vi "Projectile_Motion_2D.vi"() -> ()   [LabVIEW 2017]
panel:
  in  "Number of Particles":i32=100
  in  "Power of Force":dbl[](array[numeric])
  out "Initial Velocity":dbl[][](array[numeric])
  out "Initial Position":dbl[][](array[numeric])
  in  "Acceleration":dbl[](array[numeric])
  out "XY Graph":cluster{dbl[], dbl[]}(graph)
  in  "stop":bool
  # "IMPORTANT: The Power of force\nand the acceleration MUST be initialized\nso that the program can run. Default\nvalues for power are 1 and 1. Default\nvalues for acceleration are 0 (x direction) and\n-1 (y direction, acting like gravity).  The central\nforce term is more evident when acceleration is\nchosen to be 0 and 0 in both directions"
  # "Details: This program creates a choosen amount of\nparticles in random positions from\n-10 < position < 10 and random velocities\nfrom 0 < velocity < 1 and plots their motion. \nParticles are subjected to acceleration,\nspecular reflection once it hits a wall boundary, a \ndrag term that is veocity dependent and \na central force term whose power can be controlled by\nthe user."
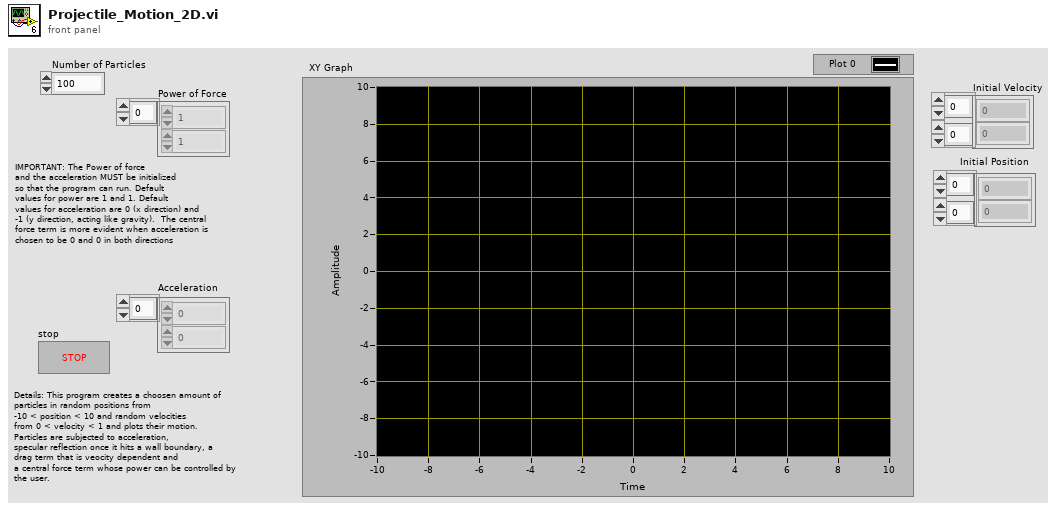
[diagram p1: front panel]
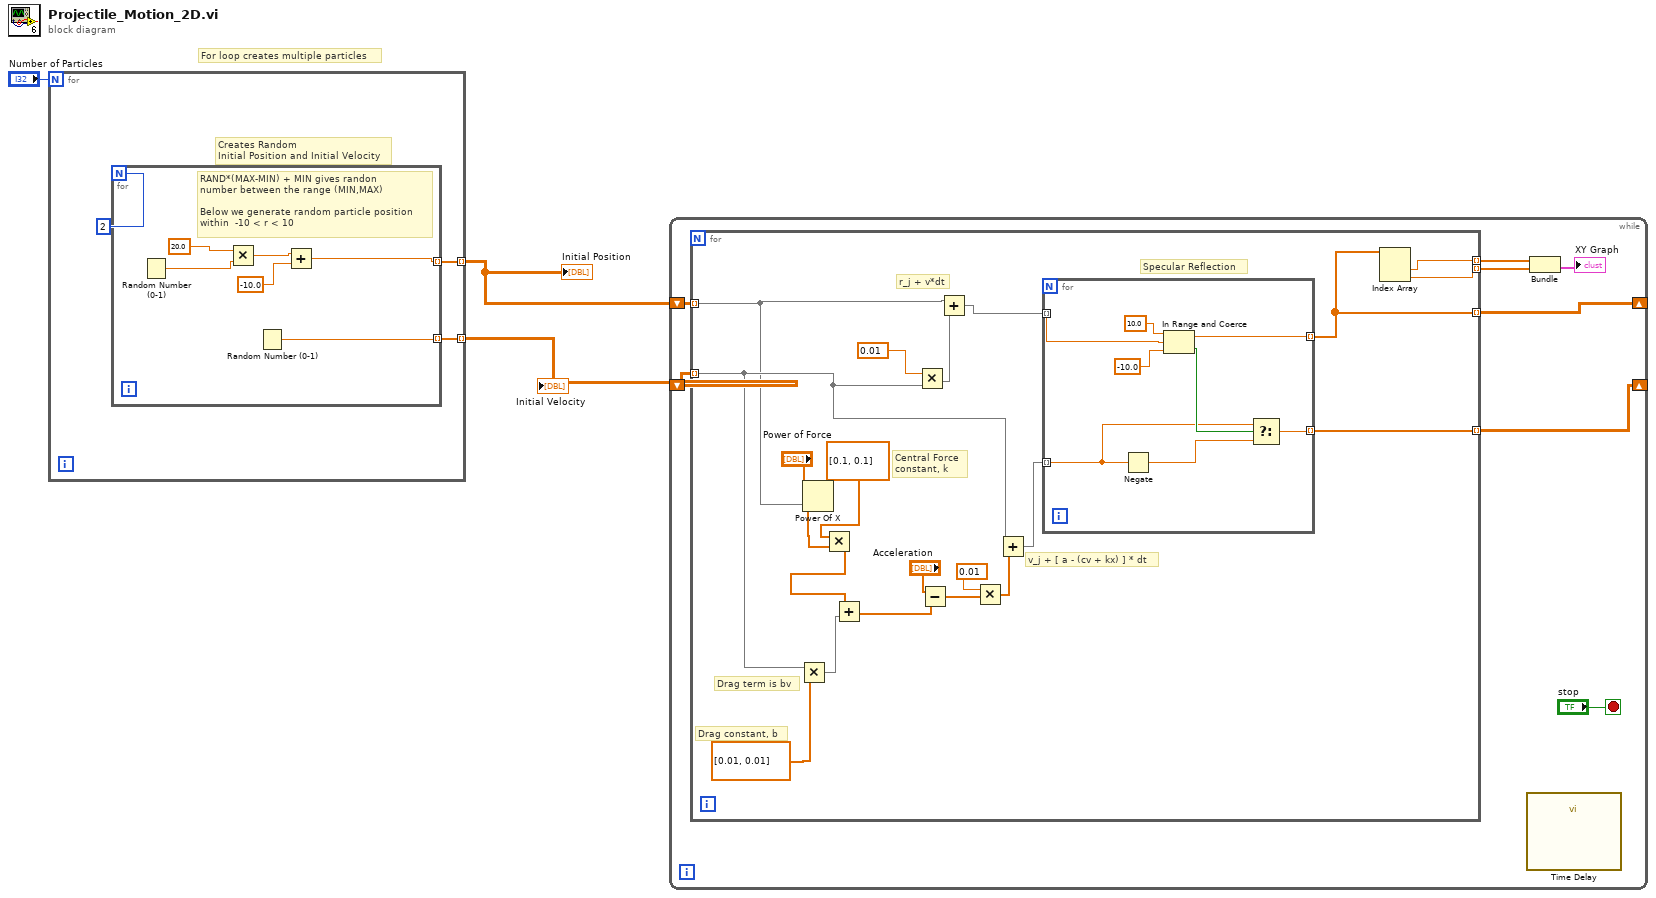
[diagram p0: block diagram]
diagram:
  # "For loop creates multiple particles"
  n1 = for {
    N: "Number of Particles" -> [_]
    tunnel: [w6] -> w3 mode=indexing
    tunnel: [w5] -> w2 mode=indexing
    # "Creates Random \nInitial Position and Initial Velocity"
    n2 = for {
      N: 2 -> [_]
      tunnel: [w12] -> w6 mode=indexing
      tunnel: [w7] -> w5 mode=indexing
      # "RAND*(MAX-MIN) + MIN gives randon\nnumber between the range (MIN,MAX)\n\nBelow we generate random particle position\nwithin  -10 < r < 10"
      n3 = Random Number (0-1)() -> (number: 0 to 1=w11:dbl)
      n4 = Multiply(x=20.0, y=w11) -> (x*y=w9:dbl)
      n5 = Random Number (0-1)() -> (number: 0 to 1=w12:dbl)
      n6 = Add(x=w9, y=-10.0) -> (x+y=w7:dbl)
    }
  }
  "Initial Position" <- w2
  "Initial Velocity" <- w3
  n7 = while {
    shift-right: [w18] -> _
    shift-left: w2 -> [w13]
    shift-right: [w17] -> _
    shift-left: w3 -> [w14]
    stop <- "stop" stop-if-true
    n8 = for {
      tunnel: [w41] -> w18 mode=indexing
      tunnel: [w40] -> w17 mode=indexing
      tunnel: [w39] -> w16 mode=indexing
      tunnel: [w38] -> w15 mode=indexing
      tunnel: w14 -> [w31] mode=indexing
      tunnel: w13 -> [w27] mode=indexing
      # "Specular Reflection"
      # "r_j + v*dt"
      # "v_j + [ a - (cv + kx) ] * dt"
      # "Central Force\nconstant, k"
      # "Drag term is bv"
      # "Drag constant, b"
      n9 = Multiply(x=w31, y=dbl[] [0.01, 0.01] ("Drag constant, b")) -> (x*y=w22:dbl[])
      n10 = Power Of X(1:w27, 2:"Power of Force") -> (0:w25:dbl[])
      n11 = Multiply(x=dbl[] [0.1, 0.1], y=w25) -> (x*y=w23:dbl[])
      n12 = Add(x=w23, y=w22) -> (x+y=w21:dbl[])
      n13 = Multiply(x=0.01, y=w31) -> (x*y=w36:dbl[])
      n14 = Subtract(x="Acceleration", y=w21) -> (x-y=w28:dbl[])
      n15 = Add(x=w27, y=w36) -> (x+y=w35:dbl[])
      n16 = Multiply(x=0.01, y=w28) -> (x*y=w33:dbl[])
      n17 = Add(x=w31, y=w33) -> (x+y=w32:dbl[])
      n18 = for {
        tunnel: w35 -> [w49] mode=indexing
        tunnel: [w46] -> w41 mode=indexing
        tunnel: w32 -> [w43] mode=indexing
        tunnel: [w42] -> w40 mode=indexing
        n19 = Negate(x=w43) -> (-x=w44:dbl)
        n20 = In Range and Coerce(upper limit=10.0, x=w49, lower limit=-10.0) -> (coerced(x)=w46:dbl, In Range?=w45:bool)
        n21 = Select(t=w43, s=w45, f=w44) -> (s? t:f=w42:dbl)
      }
      n22 = Index Array(array=w41) -> (element #1=w39:dbl, element #2=w38:dbl)  [unwired: 2 in]
    }
    n23 = call "Time Delay"() -> ()  [unwired: 11 in, 1 out]
    n24 = Bundle(w16, w15) -> (→"XY Graph":cluster{dbl[], dbl[]})  [unwired: 1 in]
  }
